vi "example.vi"() -> (0 "error out":errorcluster, 3 "VISA resource name out":refnum<visa-resource-name>)   [LabVIEW 2012, in "GPP.lvlib"]
doc: "Establishes communication with the instrument and optionally performs an instrument identification query and/or an instrument reset. It also places the instrument in a default state needed for other instrument driver operations. Therefore, call this VI before calling other instrument driver VIs for this instrument. Generally, you need to call the <B>Initialize VI</B> only once at the beginning of an application."
uses:
  GPP.lvlib
panel:
  in  "Switch":enum16{"ON", "OFF"}(ring)
  in  "Load Mode":enum16{"CV", "CC", "CR"}(ring)
  in  "OCP":enum16{"ON", "OFF"}(ring)
  in  "OVP":enum16{"ON", "OFF"}(ring)
  in  "SerialSetting":T1={"Baud Rate"=115200, "Data Bits"=8, "Parity"=0, "Stop Bits"=10} {"Stop Bits" items=["1.0"=10, "1.5"=15, "2.0"=20]; "Parity" items=["None", "Odd", "Even", "Mark", "Space"]}
  in  "Reset (True)":bool=TRUE
  in  "ID Query (True)":bool=TRUE
  in  "VISA resource name":refnum<visa-resource-name>
  out "Output State":bool
  in  "Output":bool
  in  "Beeper":bool
  in  "Track":u16(ring) items=["Indep", "Series", "Parallel"]
  out "OCP":bool
  out "OVP":bool
  out "CV/Output OFF":bool
  out "CC":bool
  out "Actual Power Level (V)":dbl format="%.3f"
  out "Mode":string
  in  "Channel  (1: CH1)":u16(ring)=1 items=["CH1"=1, "CH2"=2, "CH3"=3, "CH4"=4]
  in  "OCP  (A)":dbl format="%.3f"
  out "OCP  (A)":dbl format="%.3f"
  out "OVP  (V)":dbl format="%.3f"
  in  "OVP  (V)":dbl format="%.3f"
  in  "Current Level (A)":dbl format="%.3f"
  out "Actual Current Level (A)":dbl format="%.3f"
  out "Actual Voltage Level (V)":dbl format="%.3f"
  in  "Voltage Level (V)":dbl format="%.3f"
  # "(c) 2005-2008 National Instruments.  ALL RIGHTS RESERVED."
  # "Monitor"
  # "Settings"
  # "Protect State"
  # "Current State"
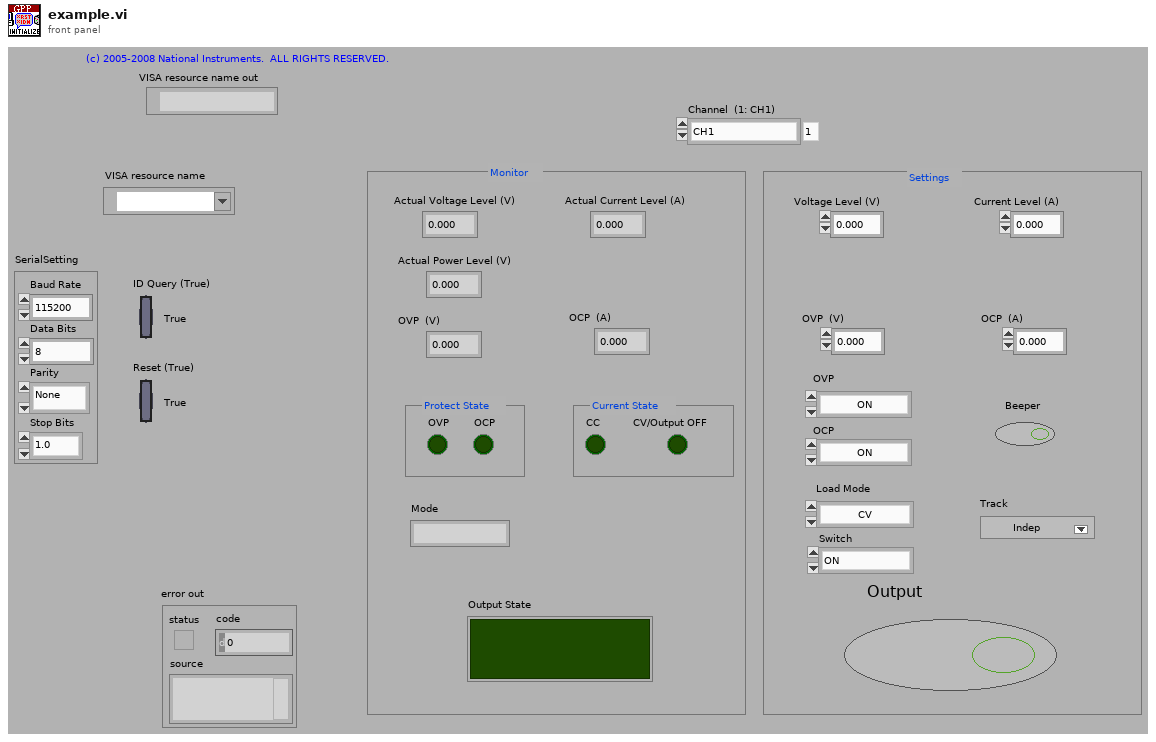
[diagram p1: front panel]
types:
  T1 = cluster{"Baud Rate":u32, "Data Bits":u16, "Parity":u16, "Stop Bits":u16}
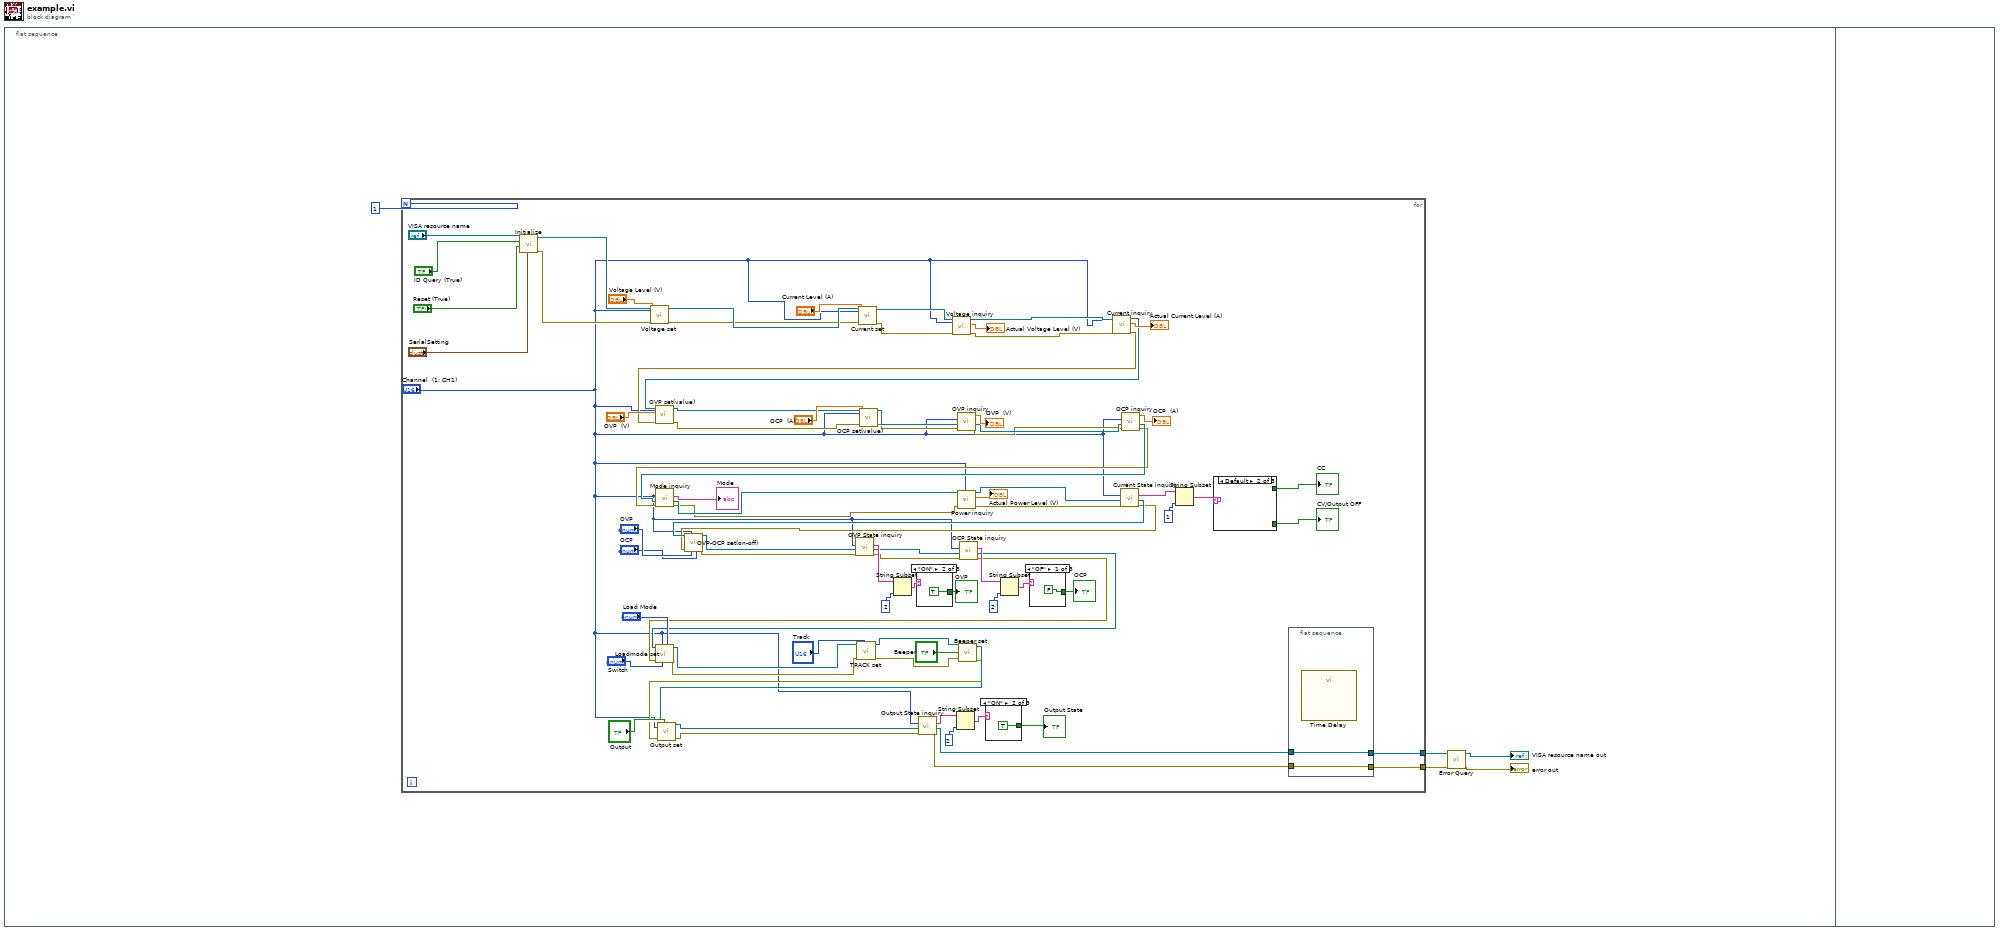
[diagram p0: block diagram]
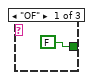
[diagram p2: hidden frame]
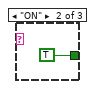
[diagram p4: hidden frame]
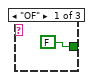
[diagram p6: hidden frame]
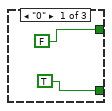
[diagram p8: hidden frame]
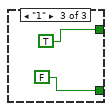
[diagram p9: hidden frame]
diagram:
  n1 = flat-sequence {
    frame #0 {
      n2 = for {
        N: 1 -> [_]
        tunnel: [w8] -> w2
        tunnel: [w6] -> w1
        n3 = call "Initialize.vi"("SerialSetting"="SerialSetting", "Reset (True)"="Reset (True)", "ID Query (True)"="ID Query (True)", "VISA resource name"="VISA resource name") -> ("error out"=w12:errorcluster, "VISA resource name out"=w11:refnum<visa-resource-name>)  [unwired: 5 in, 1 out]
        n4 = call "Voltage set.vi"("Channel  (1: CH1)"="Channel  (1: CH1)", "error in (no error)"=w12, "Voltage"="Voltage Level (V)", "VISA resource name"=w11) -> ("error out"=w49:errorcluster, "VISA resource name out"=w52:refnum<visa-resource-name>)  [unwired: 6 in]
        n5 = call "Current set.vi"("Channel  (1: CH1)"="Channel  (1: CH1)", "error in (no error)"=w49, "Current"="Current Level (A)", "VISA resource name"=w52) -> ("error out"=w48:errorcluster, "VISA resource name out"=w51:refnum<visa-resource-name>)  [unwired: 6 in]
        n6 = call "Voltage inquiry.vi"("Channel  (1: CH1)"="Channel  (1: CH1)", "error in (no error)"=w48, "VISA resource name"=w51) -> ("error out"=w47:errorcluster, "Voltage"=→"Actual Voltage Level (V)":dbl, "VISA resource name out"=w50:refnum<visa-resource-name>)  [unwired: 6 in]
        n7 = call "Current inquiry.vi"("Channel  (1: CH1)"="Channel  (1: CH1)", "error in (no error)"=w47, "VISA resource name"=w50) -> ("error out"=w45:errorcluster, "Current"=→"Actual Current Level (A)":dbl, "VISA resource name out"=w46:refnum<visa-resource-name>)  [unwired: 6 in]
        n8 = call "OVP set(value).vi"("Channel  (1: CH1)"="Channel  (1: CH1)", "error in (no error)"=w45, "OVP"="OVP  (V)", "VISA resource name"=w46) -> ("error out"=w43:errorcluster, "VISA resource name out"=w44:refnum<visa-resource-name>)  [unwired: 6 in]
        n9 = call "OCP set(value).vi"("Channel  (1: CH1)"="Channel  (1: CH1)", "error in (no error)"=w43, "OCP"="OCP  (A)", "VISA resource name"=w44) -> ("error out"=w41:errorcluster, "VISA resource name out"=w42:refnum<visa-resource-name>)  [unwired: 6 in]
        n10 = call "OVP inquiry.vi"("error in (no error)"=w41, "VISA resource name"=w42, "Channel  (1: CH1)"="Channel  (1: CH1)") -> ("error out"=w39:errorcluster, "VISA resource name out"=w40:refnum<visa-resource-name>, "OVP"=→"OVP  (V)":dbl)  [unwired: 6 in]
        n11 = call "OCP inquiry.vi"("error in (no error)"=w39, "VISA resource name"=w40, "Channel  (1: CH1)"="Channel  (1: CH1)") -> ("error out"=w37:errorcluster, "VISA resource name out"=w38:refnum<visa-resource-name>, "OCP"=→"OCP  (A)":dbl)  [unwired: 6 in]
        n12 = call "Mode inquiry.vi"("error in (no error)"=w37, "VISA resource name"=w38, "Channel  (1: CH1)"="Channel  (1: CH1)") -> ("error out"=w35:errorcluster, "VISA resource name out"=w36:refnum<visa-resource-name>, "String"=→"Mode":string)  [unwired: 6 in]
        n13 = call "Power inquiry.vi"("Channel  (1: CH1)"="Channel  (1: CH1)", "error in (no error)"=w35, "VISA resource name"=w36) -> ("error out"=w33:errorcluster, "Power"=→"Actual Power Level (V)":dbl, "VISA resource name out"=w34:refnum<visa-resource-name>)  [unwired: 6 in]
        n14 = call "Current State inquiry.vi"("error in (no error)"=w33, "VISA resource name"=w34, "Channel  (1: CH1)"="Channel  (1: CH1)") -> ("error out"=w31:errorcluster, "VISA resource name out"=w32:refnum<visa-resource-name>, "State"=w74:string)  [unwired: 6 in]
        n15 = call "OVP-OCP set(on-off).vi"("OCP"="OCP", "OVP"="OVP", "Channel  (1: CH1)"="Channel  (1: CH1)", "error in (no error)"=w31, "VISA resource in"=w32) -> ("error out"=w29:errorcluster, "VISA resource name out"=w30:refnum<visa-resource-name>)  [unwired: 5 in]
        n16 = call "OVP State inquiry.vi"("error in (no error)"=w29, "VISA resource name"=w30, "Channel  (1: CH1)"="Channel  (1: CH1)") -> ("error out"=w27:errorcluster, "VISA resource name out"=w28:refnum<visa-resource-name>, "State"=w69:string)  [unwired: 6 in]
        n17 = String Subset(string=w69, length (rest)=2) -> (substring=w67:string)  [unwired: 1 in]
        n18 = case shown="\"ON\"" w67 {
          tunnel: [FALSE TRUE _] -> w66
          frame "OF" {
          }
          frame "ON" {
          }
          frame Default {
          }
        }
        "OVP" <- w66
        n19 = call "OCP State inquiry.vi"("error in (no error)"=w27, "VISA resource name"=w28, "Channel  (1: CH1)"="Channel  (1: CH1)") -> ("error out"=w25:errorcluster, "VISA resource name out"=w26:refnum<visa-resource-name>, "State"=w68:string)  [unwired: 6 in]
        n20 = call "Loadmode set.vi"("Load Mode"="Load Mode", "Switch"="Switch", "Channel  (1: CH1)"="Channel  (1: CH1)", "error in (no error)"=w25, "VISA resource in"=w26) -> ("error out"=w23:errorcluster, "VISA resource name out"=w24:refnum<visa-resource-name>)  [unwired: 5 in]
        n21 = call "TRACK set.vi"("Track Mode"="Track", "error in (no error)"=w23, "VISA resource name"=w24) -> ("error out"=w21:errorcluster, "VISA resource name out"=w22:refnum<visa-resource-name>)  [unwired: 7 in]
        n22 = call "Beeper set.vi"("Beeper Switch (T:ON F:OFF)"="Beeper", "error in (no error)"=w21, "VISA resource in"=w22) -> ("error out"=w19:errorcluster, "VISA resource name out"=w20:refnum<visa-resource-name>)  [unwired: 7 in]
        n23 = call "Output set.vi"("Output(T:ON F:OFF)"="Output", "Channel  (1: CH1)"="Channel  (1: CH1)", "error in (no error)"=w19, "VISA resource in"=w20) -> ("error out"=w17:errorcluster, "VISA resource name out"=w18:refnum<visa-resource-name>)  [unwired: 6 in]
        n24 = call "Output State inquiry.vi"("error in (no error)"=w17, "VISA resource name"=w18, "Channel  (1: CH1)"="Channel  (1: CH1)") -> ("error out"=w7:errorcluster, "VISA resource name out"=w9:refnum<visa-resource-name>, "State"=w58:string)  [unwired: 6 in]
        n25 = String Subset(string=w58, length (rest)=2) -> (substring=w60:string)  [unwired: 1 in]
        n26 = case shown="\"ON\"" w60 {
          tunnel: [FALSE TRUE _] -> w57
          frame "OF" {
          }
          frame "ON" {
          }
          frame Default {
          }
        }
        "Output State" <- w57
        n27 = String Subset(string=w68, length (rest)=2) -> (substring=w65:string)  [unwired: 1 in]
        n28 = case shown="\"OF\"" w65 {
          tunnel: [FALSE TRUE _] -> w64
          frame "OF" {
          }
          frame "ON" {
          }
          frame Default {
          }
        }
        "OCP" <- w64
        n29 = String Subset(string=w74, length (rest)=1) -> (substring=w72:string)  [unwired: 1 in]
        n30 = case shown="Default" w72 {
          tunnel: [FALSE _ TRUE] -> w76
          tunnel: [TRUE _ FALSE] -> w75
          frame "0" {
          }
          frame Default {
          }
          frame "1" {
          }
        }
        "CC" <- w76
        "CV/Output OFF" <- w75
        n31 = flat-sequence {
          tunnel: w9 -> [w88]
          tunnel: [w88] -> w8
          tunnel: w7 -> [w87]
          tunnel: [w87] -> w6
          frame #0 {
            n32 = call "Time Delay"() -> ()  [unwired: 11 in, 1 out]
          }
        }
      }
      n33 = call "Error Query.vi"("error in (no error)"=w1, "VISA resource name"=w2) -> ("error out"=→"error out":errorcluster, "VISA resource name out"=→"VISA resource name out":refnum<visa-resource-name>)  [unwired: 6 in, 2 out]
    }
    frame #1 {
    }
  }
